vi "LVH5TCloseTypeCache.vi"(8 "error in (no error)":errorcluster, 10 "Type":enum16{"File", "Memory"}(ring), 11 "HDF5 File Ref":T1) -> (0 "error out":errorcluster, 3 "HDF5 File Ref out":T1)   [LabVIEW 2017]
doc: "LVHDF5 maintains a per-file cache of datatypes used to optimize datatype creation. This VI closes the cache associated with the file specified by id, closing all open datatypes associated with the file and committing any uncommitted datatypes to the file. This is normally called by H5Fclose.vi and, in most circumstances, does not need to be explicitly called by the user."
uses:
  <vilib>/UPVI/lvhdf5/library.llb/HDF5 Ref.ctl
panel:
  # "LVHDF5 Toolkit\nCopyright (c) 2005-2013 by Jason D. Sommerville\nCopyright (c) 2014 by UPVI, LLC.\n\nThis use and distribution of this file is governed by the terms found in \nLICENSE.txt distributed with this toolkit and installed at\n <user.lib>\\_lvhdf5\\LICENSE.txt"
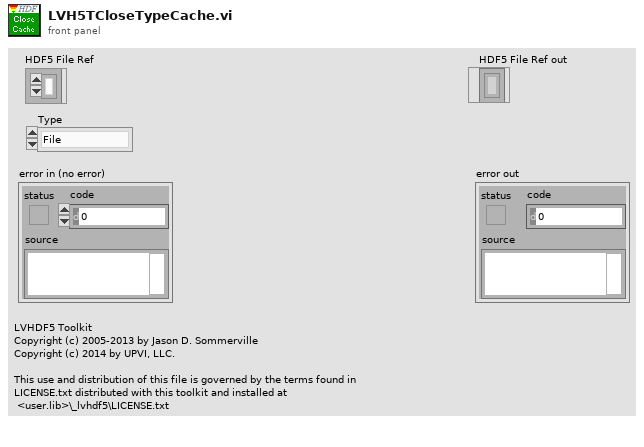
[diagram p1: front panel]
types:
  T1 = typedef "HDF5 Ref.ctl" = refnum<k1>
  T2 = enum16{"find by lvtype", "find by h5type", "index", "push", "pop", "delete last", "dequeue", "delete all"}
  T3 = typedef "LVTypeElement.ctl" = cluster{"Name":string, "TD":i16[], "Type Ref":T1, "Description":string, "Unit String":string, "Units":T4[], "Status":cluster{"MustCommit":bool, "IsCommitted":bool}}
  T4 = typedef "VariantType.lvlib/UnitInfo.ctl" = cluster{"UnitType":T5, "Exponent":i16}
  T5 = typedef "VariantType.lvlib/UnitType.ctl" = enum16{"Radians", "Steradians", "Seconds", "Meters", "Kilograms", "Amperes", "Kelvins", "Moles", "Candelas", "InvalidUnit"}
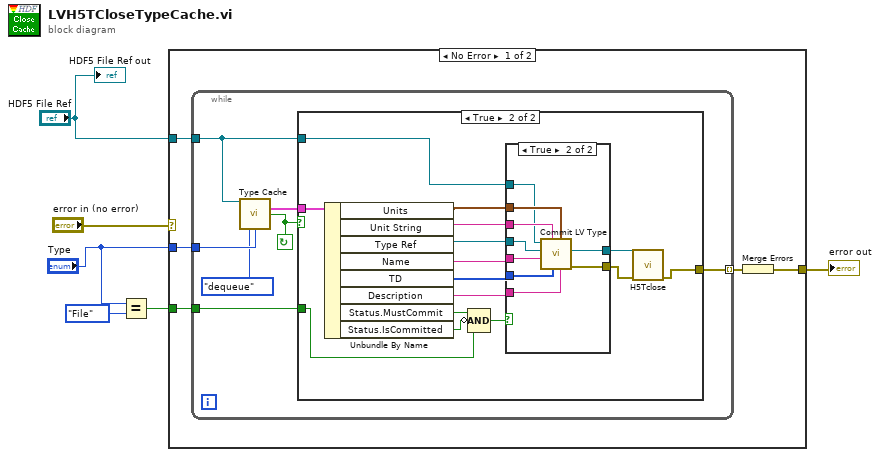
[diagram p0: block diagram]
diagram:
  n1 = Equal?(x="Type", y=enum16{"File", "Memory"}."File") -> (x = y?=w1:bool)
  n2 = case shown="No Error" "error in (no error)" {
    selector: "error in (no error)" -> [_ w44]
    tunnel: [w10 w44] -> w6
    tunnel: "HDF5 File Ref" -> [w9 _]
    tunnel: "Type" -> [w8 _]
    tunnel: w1 -> [w7 _]
    frame No Error {
      n3 = while {
        tunnel: [w16] -> w11 mode=indexing
        tunnel: w9 -> [w15]
        tunnel: w8 -> [w14]
        tunnel: w7 -> [w13]
        stop <- w18 continue-if-true
        n4 = call <vilib>:"Type Cache.vi"("HDF5  Loc Ref"=w15, "operation"=T2."dequeue", "Type"=w14) -> ("LVTypeElement out"=w17:T3, "Found?"=w18:bool)  [unwired: 9 in, 2 out]
        n5 = case shown="True" w18 {
          tunnel: w17 -> [_ w33]
          tunnel: [_ w20] -> w16
          tunnel: w15 -> [_ w23]
          tunnel: w13 -> [_ w19]
          frame False {
          }
          frame True {
            n6 = Unbundle By Name(w33) -> ("Units"=w28:T4[], "Unit String"=w29:string, "Type Ref"=w27:T1, "Name"=w26:string, "TD"=w25:i16[], "Description"=w24:string, "Status.MustCommit"=w31:bool, "Status.IsCommitted"=w32:bool)
            n7 = Compound Arithmetic op=AND(w31, invert w32, w19) -> (w30:bool)
            n8 = case shown="True" w30 {
              tunnel: w29 -> [_ w43]
              tunnel: w28 -> [_ w42]
              tunnel: w27 -> [w34 w41]
              tunnel: w26 -> [_ w40]
              tunnel: w25 -> [_ w39]
              tunnel: w24 -> [_ w38]
              tunnel: [_ w37] -> w22
              tunnel: w23 -> [_ w36]
              tunnel: [w34 w35] -> w21
              frame False {
              }
              frame True {
                n9 = call <vilib>:"Commit LV Type.vi"("Description"=w38, "Units"=w42, "Type Descriptor"=w39, "Unit String"=w43, "Name"=w40, "Type Ref"=w41, "Location Ref"=w36) -> ("error out"=w37:errorcluster, "Type Ref out"=w35:T1)  [unwired: 2 in, 1 out]
              }
            }
            n10 = call <vilib>:"H5Tclose.vi"("error in (no error)"=w22, "HDF5 Datatype Ref"=w21) -> ("error out"=w20:errorcluster)  [unwired: 7 in]
          }
        }
      }
      n11 = Merge Errors(w11) -> (w10:errorcluster)
    }
    frame Error {
    }
  }
  "error out" <- w6
  "HDF5 File Ref out" <- "HDF5 File Ref"
